vi "Set_Gain_DLPVA-100-B&F_Series.vi"(3 "error in":errorcluster, 4 "Status":i32, 5 "Gain [dB]":enum16{"20 dB", "40 dB", "60 dB", "80 dB"}(ring), 6 "index":i32) -> (0 "error out":errorcluster, 1 "Status_out":i32, 2 "index_out":i32)   [LabVIEW 2010, in "FEMTO_LUCI-10.lvlib"]
uses:
  <userlib>/FEMTO/FEMTO_LUCI-10.lvlib
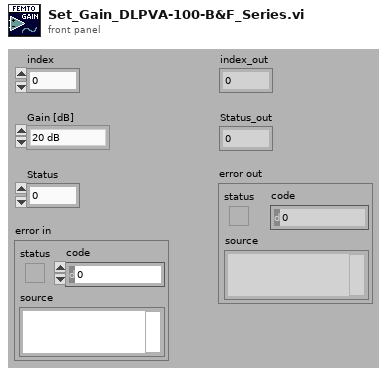
[diagram p1: front panel]
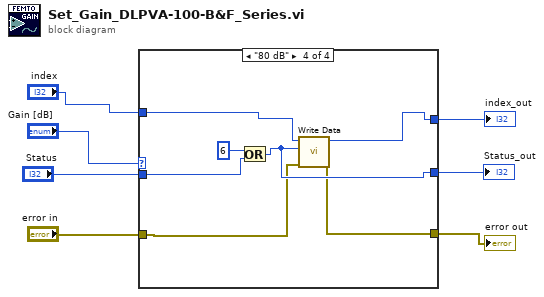
[diagram p0: block diagram]
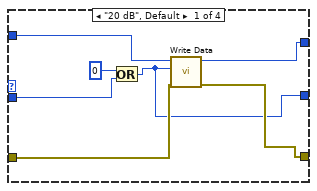
[diagram p2: hidden frame]
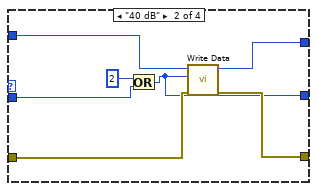
[diagram p3: hidden frame]
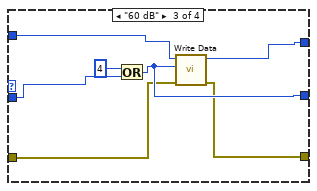
[diagram p4: hidden frame]
diagram:
  n1 = case shown="\"80 dB\"" "Gain [dB]" {
    tunnel: "index" -> [w10 w21 w27 w34]
    tunnel: [w9 w20 w26 w33] -> w2
    tunnel: "error in" -> [w12 w19 w23 w30]
    tunnel: [w11 w18 w24 w31] -> w4
    tunnel: "Status" -> [w13 w17 w22 w29]
    tunnel: [w8 w16 w25 w32] -> w6
    frame "20 dB", Default {
      n2 = Or(x=0 ("data_low"), y=w13) -> (x .or. y?=w8:i32)
      n3 = call <userlib>:"Write Data.vi"("error in (no error)"=w12, "data_low"=w8, "index"=w10) -> ("error out"=w11:errorcluster, "index_out"=w9:i32)  [unwired: 1 in, 6 out]
    }
    frame "40 dB" {
      n4 = Or(x=2 ("data_low"), y=w17) -> (x .or. y?=w16:i32)
      n5 = call <userlib>:"Write Data.vi"("error in (no error)"=w19, "data_low"=w16, "index"=w21) -> ("error out"=w18:errorcluster, "index_out"=w20:i32)  [unwired: 1 in, 6 out]
    }
    frame "60 dB" {
      n6 = Or(x=4 ("data_low"), y=w22) -> (x .or. y?=w25:i32)
      n7 = call <userlib>:"Write Data.vi"("error in (no error)"=w23, "data_low"=w25, "index"=w27) -> ("error out"=w24:errorcluster, "index_out"=w26:i32)  [unwired: 1 in, 6 out]
    }
    frame "80 dB" {
      n8 = Or(x=6 ("data_low"), y=w29) -> (x .or. y?=w32:i32)
      n9 = call <userlib>:"Write Data.vi"("error in (no error)"=w30, "data_low"=w32, "index"=w34) -> ("error out"=w31:errorcluster, "index_out"=w33:i32)  [unwired: 1 in, 6 out]
    }
  }
  "index_out" <- w2
  "error out" <- w4
  "Status_out" <- w6
